vi "Compute IK.vi"(8 "error in (no error)":errorcluster, 11 "transform":T1=[[0.43233, -0.450497, 0.781117, -0.00712862], [0.81503, -0.175371, -0.552242, -0.179284], [0.385768, 0.875384, 0.291351, 1.33346], [0.0, 0.0, 0.0, 1.0]]) -> (0 "error out":errorcluster, 2 "joints":dbl[](array[numeric]), 3 "found?":bool)   [LabVIEW 2013, in "ikfast_labview.lvlib"]
doc: "IKFAST_API bool ComputeIkC(const IkReal* eetrans, const IkReal* eerot, IkReal* joints);"
uses:
  ikfast_labview.lvlib
  <vilib>/Analysis/Matrix/Datatypes/RealMatrix.ctl
  <vilib>/robotics/Kinematics/NI_Kinematics.lvlib
  grips_labview/Telemanipulation/Grips Robot/ikfast/ikfast61.lvlib
  ikfast_labview.dll
  <vilib>/Analysis/Matrix/NI_Matrix.lvlib
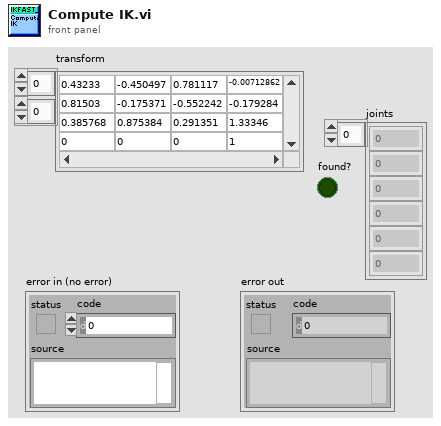
[diagram p1: front panel]
types:
  T1 = typedef "NI_Matrix.lvlib/RealMatrix.ctl" = dbl[][]
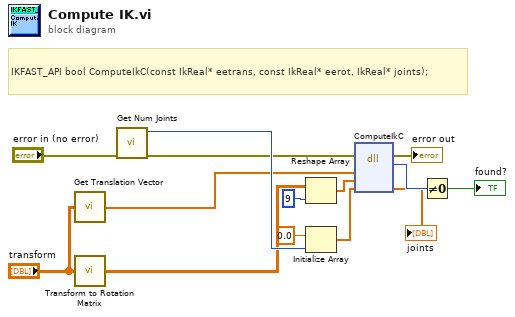
[diagram p0: block diagram]
diagram:
  # "IKFAST_API bool ComputeIkC(const IkReal* eetrans, const IkReal* eerot, IkReal* joints);"
  n1 = call <vilib>:"Get Translation Vector.vi"("transform"="transform") -> ("translation vector"=w4:dbl[])
  n2 = call <vilib>:"Transform to Rotation Matrix.vi"("transform"="transform") -> ("rotation matrix"=w2:T1)
  n3 = call "Get Num Joints.vi"("error in (no error)"="error in (no error)") -> ("error out"=w6:errorcluster, "num joints"=w8:i32)  [unwired: 9 in]
  n4 = Reshape Array(w2, 9 ("dimension size")) -> (w3:dbl[])
  n5 = Initialize Array(0.0, w8) -> (w5:dbl[])
  n6 = dll-call lib="C:/Users/fsuarez/git/ikfast_labview/user.lib/ikfast_labview/ikfast_labview.*" fn="ComputeIkC"(error in=w6, "translation"=w4, "rotation"=w3, "joints"=w5) -> (error out=→"error out":errorcluster, "return type"=w13:u8, "joints"=→"joints":dbl[])  [unwired: 4 in, 1 out]
  n7 = Not Equal To 0?(x=w13) -> (x != 0?=→"found?":bool)
